vi "Parse Data JSON.vi"(8 "error in (no error)":errorcluster, 10 "JSON String":string, 11 "Identified in":refnum<class "Identified.lvclass">) -> (0 "error out":errorcluster, 1 "Typed?":bool, 2 "Typed Message":refnum<class "Response.lvclass">, 3 "Identified out":refnum<class "Identified.lvclass">)   [LabVIEW 2022 SP3, in "obs-websocket-lv.lvlib" / "Identified.lvclass"]
uses:
  Identified.lvclass
  Identified.lvclass/Identified.ctl
  <vilib>/IlluminatedG/lv-web-crypto/lv-json/JSON/JSON.lvlib
  Response/Response.lvclass
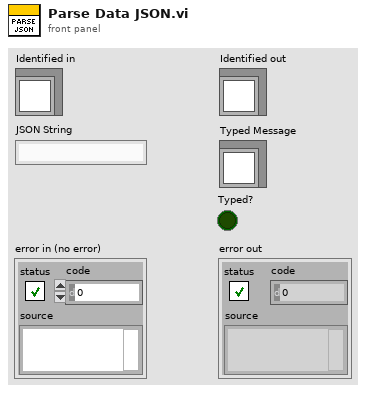
[diagram p1: front panel]
types:
  T1 = typedef "JSON.lvlib/JSON Item Type.ctl" = enum16{"unknown", "null", "Array", "Object", "String", "Number", "Boolean"}
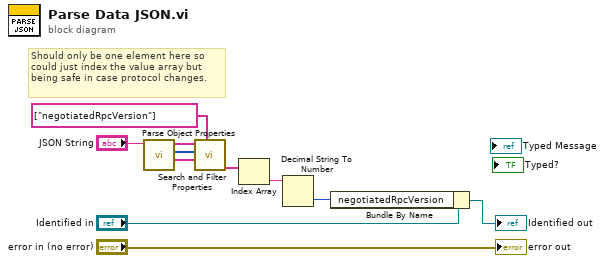
[diagram p0: block diagram]
diagram:
  # "Should only be one element here so could just index the value array but being safe in case protocol changes."
  n1 = call <vilib>:"Parse Object Properties.vi"("JSON String"="JSON String") -> ("Values"=w6:string[], "Item Types"=w7:T1[], "Keys"=w8:string[])  [unwired: 7 in, 1 out]
  n2 = call <vilib>:"Search and Filter Properties.vi"("Search Keys"=string[] ["negotiatedRpcVersion"], "Values In"=w6, "Types In"=w7, "Keys In"=w8) -> ("Filtered Values"=w4:string[])  [unwired: 2 in, 5 out]
  n3 = Index Array(array=w4) -> (element=w3:string)  [unwired: 1 in]
  n4 = Decimal String To Number(string=w3) -> (number=w1:i32)  [unwired: 2 in, 1 out]
  n5 = Bundle By Name(cluster="Identified in", "negotiatedRpcVersion"=w1) -> (→"Identified out":refnum<class "Identified.lvclass">)
  "error out" <- "error in (no error)"
